vi "Doppler.vi"() -> ()   [LabVIEW 2020]
uses:
  <vilib>/Analysis/3filter.llb/Filter Passband Type.ctl
  <vilib>/Analysis/5stat.llb/RMS (DBL).vi
  <vilib>/Analysis/3filter.llb/Butterworth Filter (DBL).vi
  <vilib>/Analysis/NI_AALBase.lvlib
  <vilib>/Analysis/NI_AALPro.lvlib
  <vilib>/measure/NI_MABase.lvlib
panel:
  in  "phase":dbl format="%.2p"
  out "Signal In":waveform(dbl)(graph)
  out "Filtered X":dbl[](array[numeric])
  in  "fl":dbl=0.12500000000000006 format="%0.4f"
  in  "fh":dbl=0.45000000000000007 format="%0.2f"
  in  "fs":dbl=1.0 format="%0.2f"
  out "RMS value (V)":dbl format="%0.2f"
  out "Signal Out":dbl[](graph)
  in  "Stop":bool
  out "Center_Frequency":dbl
  in  "v":dbl
  in  "Amplitude":dbl=1.0
  in  "Frequency":dbl=1000.0
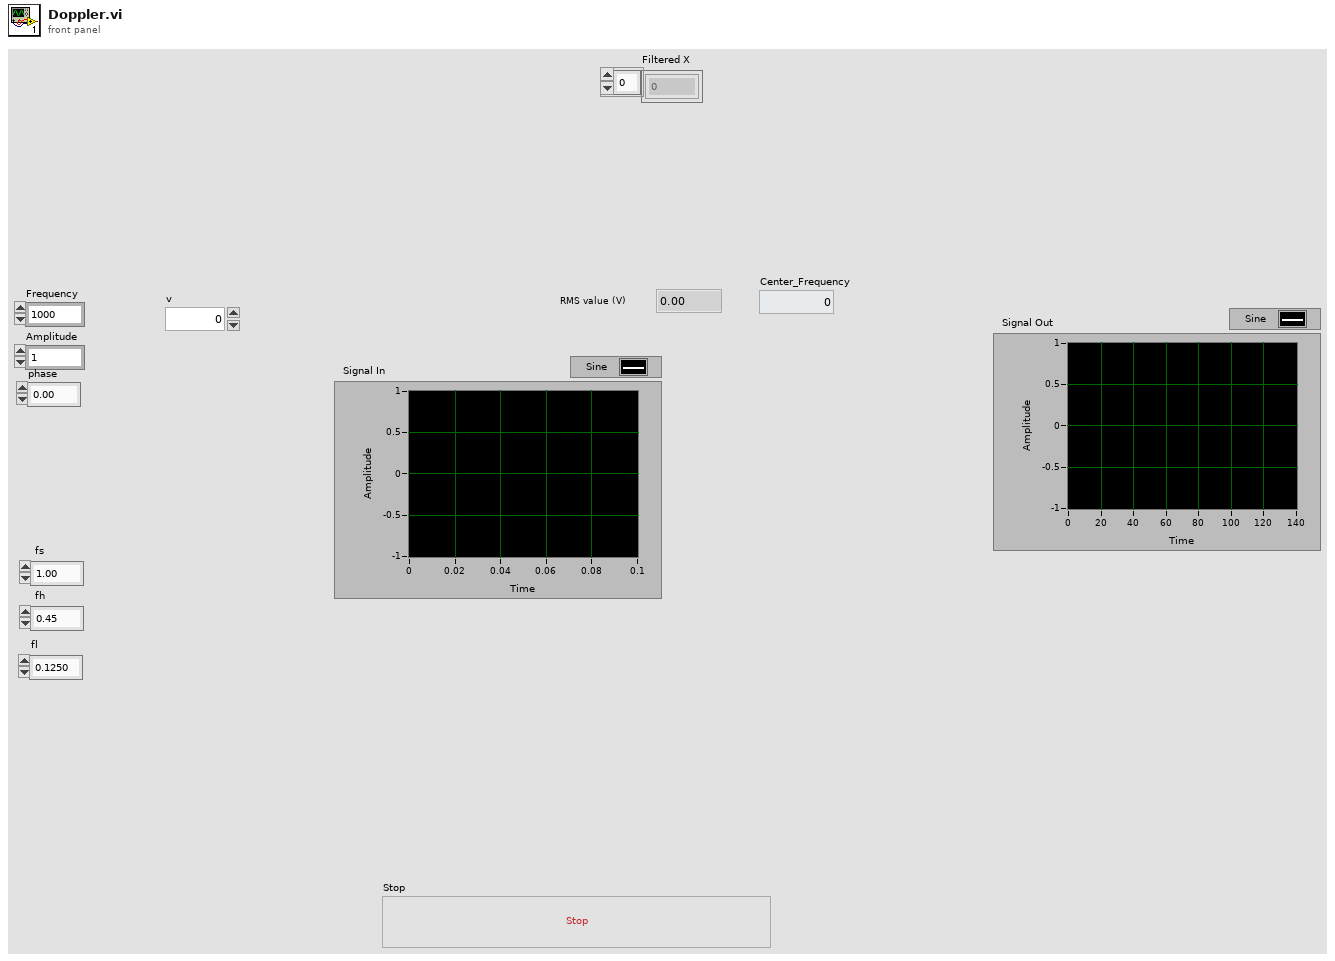
[diagram p1: front panel]
types:
  T1 = typedef "NI_AALBase.lvlib/Filter Passband Type.ctl" = enum32{"Lowpass", "Highpass", "Bandpass", "Bandstop"}
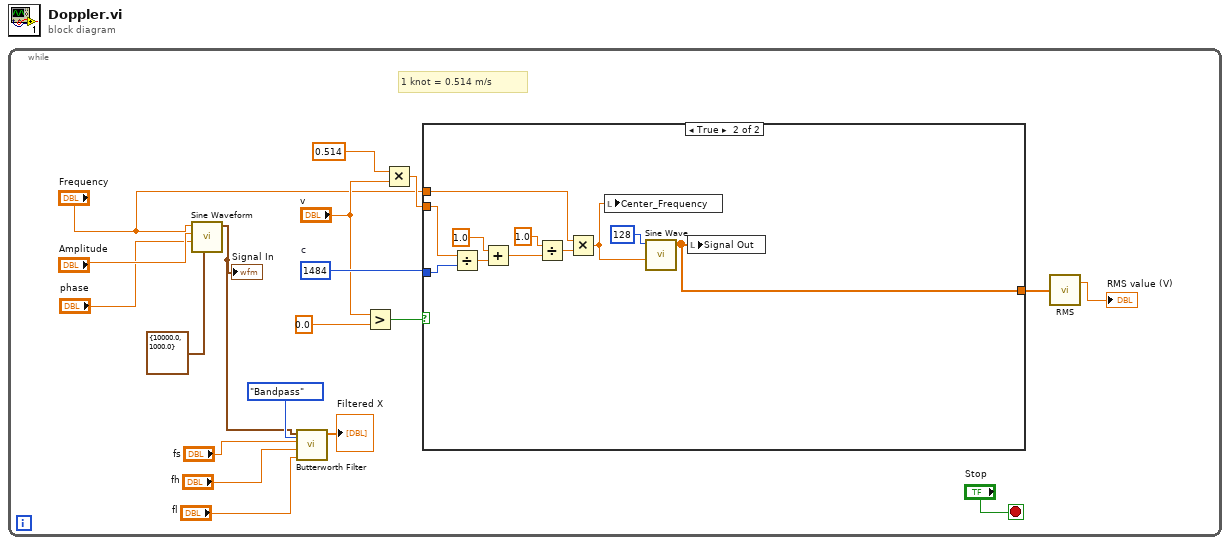
[diagram p0: block diagram]
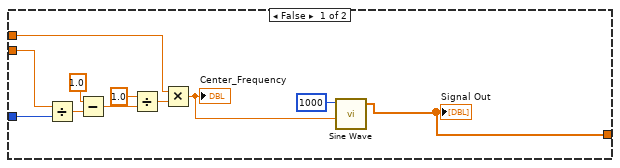
[diagram p2: hidden frame]
diagram:
  n1 = while {
    stop <- "Stop" stop-if-true
    w17 = 1484  # c
    # "1 knot = 0.514 m/s"
    n2 = call <vilib>:"Sine Waveform.vi"("sampling info"=cluster{"Fs":dbl, "#s":dbl} {"Fs"=10000.0, "#s"=1000.0}, "phase"="phase", "amplitude"="Amplitude", "frequency"="Frequency") -> ("signal out"=w1:waveform(dbl))  [unwired: 6 in, 1 out]
    "Signal In" <- w1
    n3 = call-poly <vilib>:"Butterworth Filter.vi"("filter type"=Filter_Passband_Type."Bandpass", "low cutoff freq: fl"="fl", "high cutoff freq: fh"="fh", "sampling freq: fs"="fs", "X"=w1) -> ("Filtered X"=→"Filtered X":dbl[])  [unwired: 3 in, 1 out]
    n4 = Greater?(x="v", y=0.0) -> (0:w18:bool)
    n5 = Multiply(x=0.514 ("y"), y="v") -> (x*y=w13:dbl)
    n6 = case shown="True" w18 {
      tunnel: "Frequency" -> [w26 w41]
      tunnel: w13 -> [w27 w40]
      tunnel: w17 -> [w28 w39]
      tunnel: [w20 w31] -> w3
      frame False {
        n7 = Divide(x=w27, y=w28) -> (x/y=w24:dbl)
        n8 = Subtract(x=1.0 ("y"), y=w24) -> (x-y=w23:dbl)
        n9 = Divide(x=1.0, y=w23) -> (x/y=w29:dbl)
        n10 = Multiply(x=w26, y=w29) -> (x*y=w22:dbl)
        "Center_Frequency" <- w22
        n11 = call <vilib>:"Sine Wave.vi"("samples"=1000, "frequency"=w22) -> ("sine wave"=w20:dbl[])  [unwired: 3 in, 2 out]
        "Signal Out" <- w20
      }
      frame True {
        n12 = Divide(x=w40, y=w39) -> (x/y=w34:dbl)
        n13 = Add(x=1.0 ("y"), y=w34) -> (x+y=w38:dbl)
        n14 = Divide(x=1.0, y=w38) -> (x/y=w36:dbl)
        n15 = Multiply(x=w41, y=w36) -> (x*y=w32:dbl)
        n16 = local write "Center_Frequency"(w32) -> ()
        n17 = call <vilib>:"Sine Wave.vi"("samples"=128, "frequency"=w32) -> ("sine wave"=w31:dbl[])  [unwired: 3 in, 2 out]
        n18 = local write "Signal Out"(w31) -> ()
      }
    }
    n19 = call-poly <vilib>:"RMS.vi"("X"=w3) -> ("rms value"=→"RMS value (V)":dbl)  [unwired: 1 out]
  }
